vi "ReadBitS0_32.vi"(7 "error in (no error)":errorcluster, 8 "BitAddr":u8, 9 "address":u32) -> (0 "error out":errorcluster, 3 "Bool Board 1":bool)   [LabVIEW 2015, in "ESLSCDLL.lvlib"]
uses:
  ESLSCDLL.lvlib
  Globals.vi
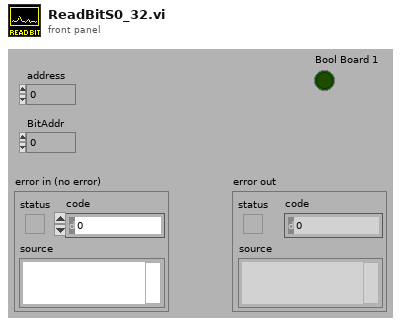
[diagram p1: front panel]
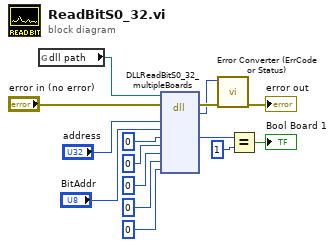
[diagram p0: block diagram]
diagram:
  n1 = global read "Globals.vi" "dll path"() -> (w1:path)
  n2 = dll-call lib="C:/ENTW/PCIE/LV64/board.vis/ESLSCDLL.dll" fn="DLLReadBitS0_32_multipleBoards" ("lwlscdll.dll:DLLReadLongS0")(path in=w1, error in="error in (no error)", "address"="address", "bitnumber"="BitAddr", "isBitHigh0"=u32 0 ("data"), "isBitHigh1"=u32 0 ("data1"), "isBitHigh2"=u32 0 ("data2"), "isBitHigh3"=u32 0 ("data3"), "isBitHigh4"=u32 0 ("data4")) -> (error out=w13:errorcluster, "es_status_codes"=w12:i32, "isBitHigh0"=w3:u32)  [unwired: 7 in, 1 out]
  n3 = call "Error Converter (ErrCode or Status).vi"("error in (no error)"=w13, "error code"=w12) -> ("error out"=→"error out":errorcluster)  [unwired: 9 in]
  n4 = Equal?(x=w3, y=u32 1) -> (x = y?=→"Bool Board 1":bool)
